vi "vi.GetTypeName.vi"(0 "Type Descriptor":i16[](array[numeric]), 11 "error in":errorcluster) -> (4 "Name":string, 15 "error out":errorcluster)   [LabVIEW 2014, in "GLue.lvlib" / "class.GLue.lvclass"]
uses:
  class.GLue.lvclass
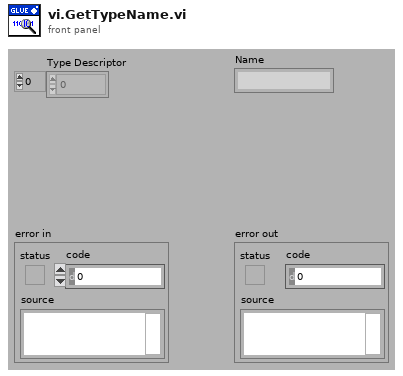
[diagram p1: front panel]
types:
  T1 = cluster{"length":u16, "private":u8, "type":enum8{"<Null>", "I8", "I16", "I32", "I64", "U8", "U16", "U32", "U64", "SGL", "DBL", "EXT", "CSG", "CDB", "CXT", "0x0F", "0x10", "0x11", "0x12", "0x13", "0x14", "Enum U8", "Enum U16", "Enum U32", "Enum U64", "SGL PQ", "DBL PQ", "EXT PQ", "CSG PQ", "CDB PQ", "CXT PQ", "0x1F", "0x20", "Boolean", "0x22", "0x23", "0x24", "0x25", "0x26", "0x27", "0x28", "0x29", "0x2A", "0x2B", "0x2C", "0x2D", "0x2E", "0x2F", "String", "0x31", "Path", "Pict", "0x34", "0x35", "0x36", "DAQ", "0x38", "0x39", "0x3A", "0x3B", "0x3C", "0x3D", "0x3E", "0x3F", "Array", "0x41", "0x42", "0x43", "0x44", "0x45", "0x46", "0x47", "0x48", "0x49", "0x4A", "0x4B", "0x4C", "0x4D", "0x4E", "0x4F", "Cluster", "0x51", "0x52", "Variant", "Waveform", "0x55", "0x56", "0x57", "0x58", "0x59", "0x5A", "0x5B", "0x5C", "0x5D", "0x5E", "0x5F", "0x60", "0x61", "0x62", "0x63", "0x64", "0x65", "0x66", "0x67", "0x68", "0x69", "0x6A", "0x6B", "0x6C", "0x6D", "0x6E", "0x6F", "Refnum"}, "# elements":u16}
  T2 = enum8{"<Null>", "I8", "I16", "I32", "I64", "U8", "U16", "U32", "U64", "SGL", "DBL", "EXT", "CSG", "CDB", "CXT", "0x0F", "0x10", "0x11", "0x12", "0x13", "0x14", "Enum U8", "Enum U16", "Enum U32", "Enum U64", "SGL PQ", "DBL PQ", "EXT PQ", "CSG PQ", "CDB PQ", "CXT PQ", "0x1F", "0x20", "Boolean", "0x22", "0x23", "0x24", "0x25", "0x26", "0x27", "0x28", "0x29", "0x2A", "0x2B", "0x2C", "0x2D", "0x2E", "0x2F", "String", "0x31", "Path", "Pict", "0x34", "0x35", "0x36", "DAQ", "0x38", "0x39", "0x3A", "0x3B", "0x3C", "0x3D", "0x3E", "0x3F", "Array", "0x41", "0x42", "0x43", "0x44", "0x45", "0x46", "0x47", "0x48", "0x49", "0x4A", "0x4B", "0x4C", "0x4D", "0x4E", "0x4F", "Cluster", "0x51", "0x52", "Variant", "Waveform", "0x55", "0x56", "0x57", "0x58", "0x59", "0x5A", "0x5B", "0x5C", "0x5D", "0x5E", "0x5F", "0x60", "0x61", "0x62", "0x63", "0x64", "0x65", "0x66", "0x67", "0x68", "0x69", "0x6A", "0x6B", "0x6C", "0x6D", "0x6E", "0x6F", "Refnum"}
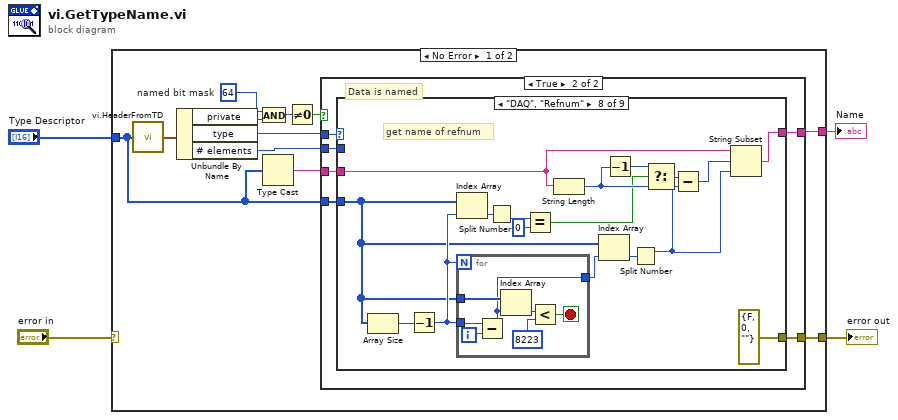
[diagram p0: block diagram]
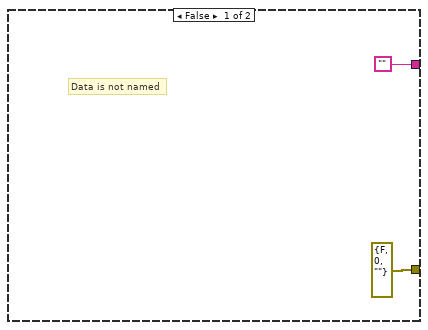
[diagram p2: hidden frame]
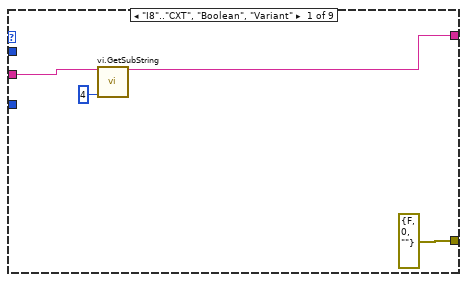
[diagram p3: hidden frame]
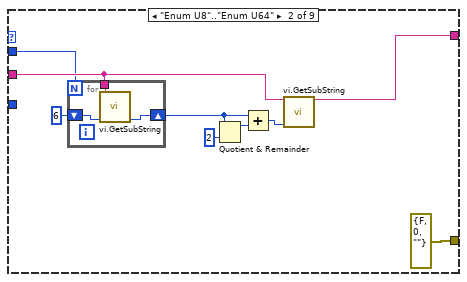
[diagram p4: hidden frame]
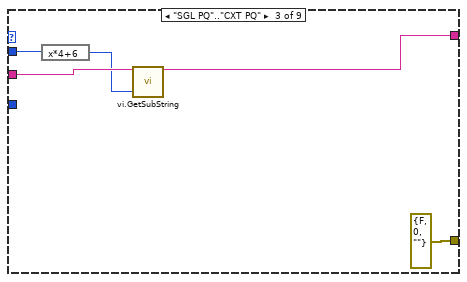
[diagram p5: hidden frame]
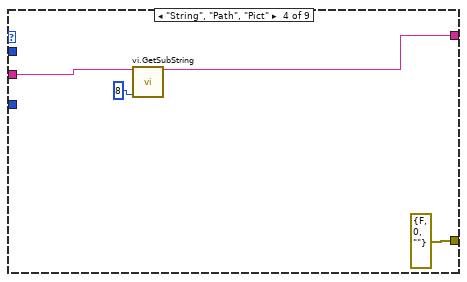
[diagram p6: hidden frame]
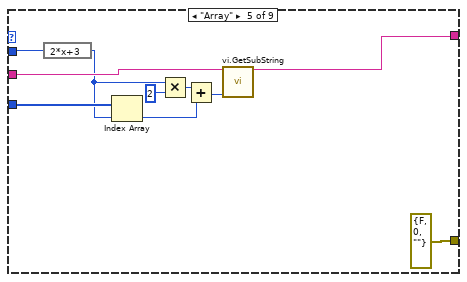
[diagram p7: hidden frame]
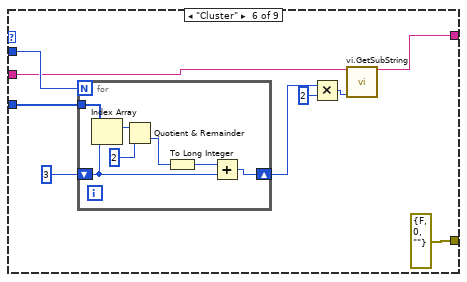
[diagram p8: hidden frame]
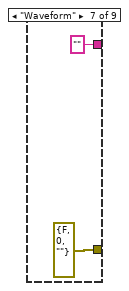
[diagram p9: hidden frame]
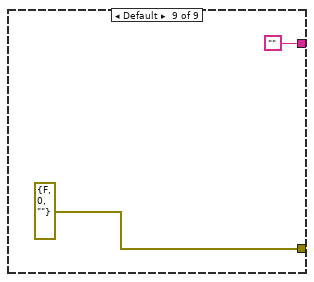
[diagram p10: hidden frame]
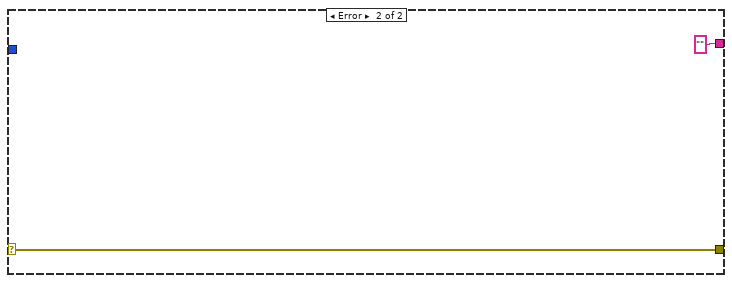
[diagram p11: hidden frame]
diagram:
  n1 = case shown="No Error" "error in" {
    selector: "error in" -> [_ w104]
    tunnel: [w13 "" ("Last PString")] -> w1
    tunnel: [w7 w104] -> w2
    tunnel: "Type Descriptor" -> [w5 _]
    frame No Error {
      w10 = u8 64  # named bit mask
      n2 = call "vi.HeaderFromTD.vi"("Type Descriptor"=w5) -> ("Type Descriptor Header"=w6:T1)  [unwired: 4 in]
      n3 = Unbundle By Name(w6) -> ("private"=w9:u8, "type"=w8:T2, "# elements"=w15:u16)
      n4 = And(x=w10, y=w9) -> (x .and. y?=w12:u8)
      n5 = Type Cast(x=w5) -> (*(type *) &x=w14:string)  [unwired: 1 in]
      n6 = Not Equal To 0?(x=w12) -> (x != 0?=w11:bool)
      n7 = case shown="True" w11 {
        tunnel: [errorcluster {"status"=FALSE, "code"=0, "source"=""} ("error out") w23] -> w7
        tunnel: w8 -> [_ w22]
        tunnel: w14 -> [_ w21]
        tunnel: ["" w20] -> w13
        tunnel: w15 -> [_ w19]
        tunnel: w5 -> [_ w18]
        frame False {
          # "Data is not named"
        }
        frame True {
          # "Data is named"
          n8 = case shown="\"DAQ\", \"Refnum\"" w22 {
            tunnel: [errorcluster {"status"=FALSE, "code"=0, "source"=""} ("error out") errorcluster {"status"=FALSE, "code"=0, "source"=""} ("error out") errorcluster {"status"=FALSE, "code"=0, "source"=""} ("error out") errorcluster {"status"=FALSE, "code"=0, "source"=""} ("error out") errorcluster {"status"=FALSE, "code"=0, "source"=""} ("error out") errorcluster {"status"=FALSE, "code"=0, "source"=""} ("error out") errorcluster {"status"=FALSE, "code"=0, "source"=""} ("error out") errorcluster {"status"=FALSE, "code"=0, "source"=""} ("error out") errorcluster {"status"=FALSE, "code"=0, "source"=""} ("error out")] -> w23
            tunnel: w21 -> [w26 w33 w43 w48 w55 w64 _ w80 _]
            tunnel: [w24 w32 w41 w47 w54 w63 "" ("Last PString") w81 ""] -> w20
            tunnel: w19 -> [_ w30 w44 _ w57 w66 _ _ _]
            tunnel: w18 -> [_ _ _ _ w56 w65 _ w86 _]
            frame "I8".."CXT", "Boolean", "Variant" {
              n9 = call "vi.GetSubString.vi"("String"=w26, "offset (0)"=4) -> ("SubString"=w24:string)  [unwired: 12 in, 1 out]
            }
            frame "Enum U8".."Enum U64" {
              n10 = for {
                N: w30 -> [_]
                tunnel: w33 -> [w37]
                shift-right: [w38] -> w35
                shift-left: 6 -> [w39]
                n11 = call "vi.GetSubString.vi"("String"=w37, "offset (0)"=w39) -> ("offset past SubString"=w38:i32)  [unwired: 12 in, 1 out]
              }
              n12 = Quotient & Remainder(x=w35, y=2) -> (x-y*floor(x/y)=w28:i32)  [unwired: 1 out]
              n13 = Add(x=w35, y=w28) -> (x+y=w34:i32)
              n14 = call "vi.GetSubString.vi"("String"=w33, "offset (0)"=w34) -> ("SubString"=w32:string)  [unwired: 12 in, 1 out]
            }
            frame "SGL PQ".."CXT PQ" {
              n15 = expression code="x*4+6"(w44) -> (w42:u16)
              n16 = call "vi.GetSubString.vi"("String"=w43, "offset (0)"=w42) -> ("SubString"=w41:string)  [unwired: 12 in, 1 out]
            }
            frame "String", "Path", "Pict" {
              n17 = call "vi.GetSubString.vi"("String"=w48, "offset (0)"=8) -> ("SubString"=w47:string)  [unwired: 12 in, 1 out]
            }
            frame "Array" {
              n18 = expression code="2*x+3"(w57) -> (w53:u16)
              n19 = Index Array(array=w56, index=w53) -> (element=w50:i16)
              n20 = Multiply(x=w53, y=u16 2) -> (x*y=w51:u16)
              n21 = Add(x=w51, y=w50) -> (x+y=w49:u16)
              n22 = call "vi.GetSubString.vi"("String"=w55, "offset (0)"=w49) -> ("SubString"=w54:string)  [unwired: 12 in, 1 out]
            }
            frame "Cluster" {
              n23 = for {
                N: w66 -> [_]
                shift-right: [w73] -> w61
                shift-left: 3 -> [w72]
                tunnel: w65 -> [w74]
                n24 = Index Array(array=w74, index=w72) -> (element=w70:i16)
                n25 = Quotient & Remainder(x=w70, y=i16 2) -> (floor(x/y)=w71:i16)  [unwired: 1 out]
                n26 = To Long Integer(number=w71) -> (32bit integer=w68:i32)
                n27 = Add(x=w68, y=w72) -> (x+y=w73:i32)
              }
              n28 = Multiply(x=w61, y=2) -> (x*y=w60:i32)
              n29 = call "vi.GetSubString.vi"("String"=w64, "offset (0)"=w60) -> ("SubString"=w63:string)  [unwired: 12 in, 1 out]
            }
            frame "Waveform" {
            }
            frame "DAQ", "Refnum" {
              # "get name of refnum"
              n30 = Array Size(array=w86) -> (size(s)=w92:i32)
              n31 = Decrement(x=w92) -> (x-1=w88:i32)
              n32 = Index Array(array=w86, index=w88) -> (element=w89:i16)
              n33 = for {
                N: w88 -> [_]
                tunnel: w88 -> [w99]
                tunnel: w86 -> [w100]
                tunnel: [w95] -> w85
                i -> [w98]
                stop <- w96 stop-if-true
                n34 = Subtract(x=w99, y=w98) -> (x-y=w95:i32)
                n35 = Index Array(array=w100, index=w95) -> (element=w94:i16)
                n36 = Less?(x=w94, y=i16 8223) -> (x < y?=w96:bool)
              }
              n37 = Split Number(x=w89) -> (lo(x)=w90:u8)  [unwired: 1 out]
              n38 = Equal?(x=w90, y=u8 0) -> (x = y?=w82:bool)
              n39 = String Length(string=w80) -> (length=w84:i32)
              n40 = Index Array(array=w86, index=w85) -> (element=w87:i16)
              n41 = Decrement(x=w84) -> (x-1=w83:i32)
              n42 = Split Number(x=w87) -> (hi(x)=w77:u8)  [unwired: 1 out]
              n43 = Select(t=w83, s=w82, f=w84) -> (s? t:f=w79:i32)
              n44 = Subtract(x=w79, y=w77) -> (x-y=w78:i32)
              n45 = String Subset(string=w80, offset (0)=w78, length (rest)=w77) -> (substring=w81:string)
            }
            frame Default {
            }
          }
        }
      }
    }
    frame Error {
    }
  }
  "error out" <- w2
  "Name" <- w1
